vi "3D_box.vi"(8 "PITCH":dbl, 9 "ROLL":dbl, 11 "Color":u32(colorbox)) -> (3 "3D Picture":refnum<vi>(3d-picture))   [LabVIEW 2025]
uses:
  <vilib>/picture/3D Picture Control/Object/Add Object (no reference).vi
  <vilib>/picture/3D Picture Control/Object/Create Object (name).vi
  <vilib>/picture/3D Picture Control/NI_3D Picture Control.lvlib
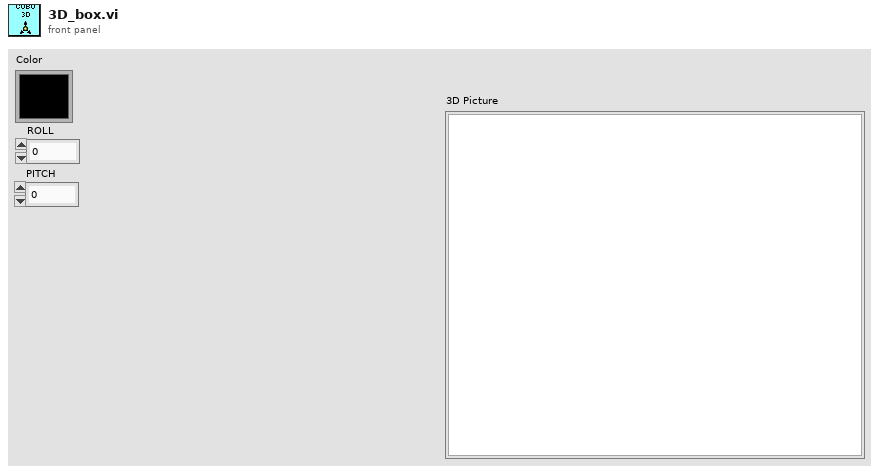
[diagram p1: front panel]
types:
  T1 = cluster{"Red":sgl, "Green":sgl, "Blue":sgl, "Alpha":sgl}
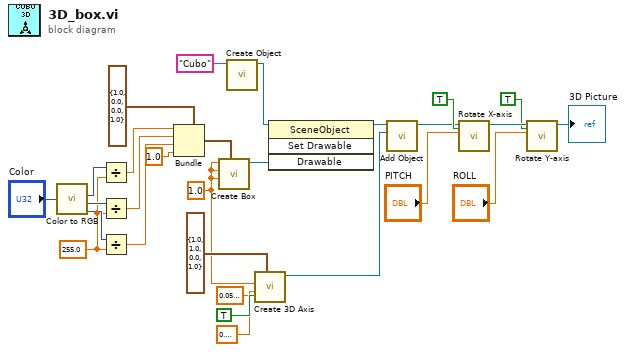
[diagram p0: block diagram]
diagram:
  w3 = sgl 1.0 ("Alpha")
  w19 = sgl 255.0 ("Alpha")
  n1 = call <vilib>:"Color to RGB.vi"("Color"="Color") -> ("R"=w22:u8, "G"=w21:u8, "B"=w20:u8)  [unwired: 1 out]
  n2 = Divide(x=w22, y=w19) -> (x/y=w18:sgl)
  n3 = Divide(x=w21, y=w19) -> (x/y=w17:sgl)
  n4 = Divide(x=w20, y=w19) -> (x/y=w16:sgl)
  n5 = Bundle(cluster=T1 {"Red"=1.0, "Green"=0.0, "Blue"=0.0, "Alpha"=1.0} ("Color"), "Red"=w18, "Green"=w17, "Blue"=w16, "Alpha"=sgl 1.0) -> (w23:T1)
  n6 = call <vilib>:"Create Box.vi"("Color"=w23, "Length Z"=w3, "Length Y"=w3, "Length X"=w3) -> ("New Box Refnum"=w27:refnum<vi>)  [unwired: 6 in, 1 out]
  n7 = call-poly <vilib>:"Create Object.vi"("Name"="Cubo") -> ("Scene:New Object"=w28:refnum<vi>)  [unwired: 9 in, 1 out]
  n8 = call <vilib>:"Create 3D Axis.vi"("Character Size"=sgl 0.3 ("Alpha"), "Axis label?"=TRUE, "Color"=T1 {"Red"=1.0, "Green"=1.0, "Blue"=0.0, "Alpha"=1.0}, "Radius"=sgl 0.05 ("Alpha"), "Length"=w3) -> ("New Object Refnum"=w9:refnum<vi>)  [unwired: 5 in, 1 out]
  n9 = invoke class="SceneObject" method="Set Drawable"(reference=w28, "Drawable"=w27) -> (reference out=w10:refnum<vi>)  [unwired: 2 in, 3 out]
  n10 = call-poly <vilib>:"Add Object.vi"("New Object In"=w9, "Scene Object In"=w10) -> ("Scene Object Out"=w1:refnum<vi>)  [unwired: 8 in, 1 out]
  n11 = call <vilib>:"Rotate X-axis.vi"("Relative?"=TRUE, "angle"="PITCH", "Scene Object In"=w1) -> ("Scene Object Out"=w15:refnum<vi>)  [unwired: 7 in, 1 out]
  n12 = call <vilib>:"Rotate Y-axis.vi"("Relative?"=TRUE, "angle"="ROLL", "Scene Object In"=w15) -> ("Scene Object Out"=→"3D Picture":refnum<vi>)  [unwired: 7 in, 1 out]
